vi "Subpanel - Load VI.vi"(7 "SubPanel in":refnum<vi>, 8 "error in (no error)":errorcluster, 10 "VI Reference":refnum<vi>, 11 "Subpanel VI Ref IN":refnum<vi>) -> (0 "error out":errorcluster, 2 "Removed Module":string, 3 "Subpanel VI Ref OUT":refnum<vi>)   [LabVIEW 2022 SP3, in "hse-ui.lvlib"]
doc: "Opens the VI reference to <b>Full Delimited Name</b> and inserts it into <b>SubPanel in</b>. The reference of the inserted VI is returned in Subpanel VI Ref OUT.\n\nIf Subpanel VI Ref IN is a valid reference, the front panel of the referenced VI is opened hidden before removing it from the subpanel in order to avoid losing the VI from memory.\n\n____\nHAMPEL SOFTWARE ENGINEERING v3.8.0 (2023-12-18 14:41)"
uses:
  hse-ui.lvlib
  hse-dqmh/hse-dqmh.lvlib
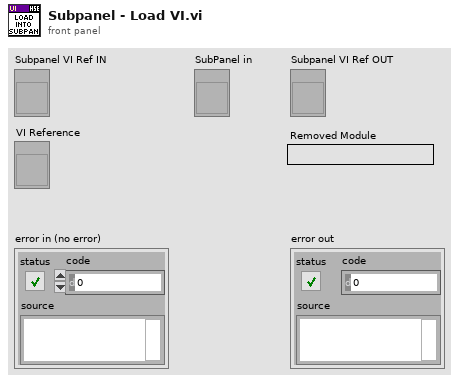
[diagram p1: front panel]
types:
  T1 = enum32{"Invalid", "Standard", "Closed", "Hidden", "Minimized", "Maximized"}
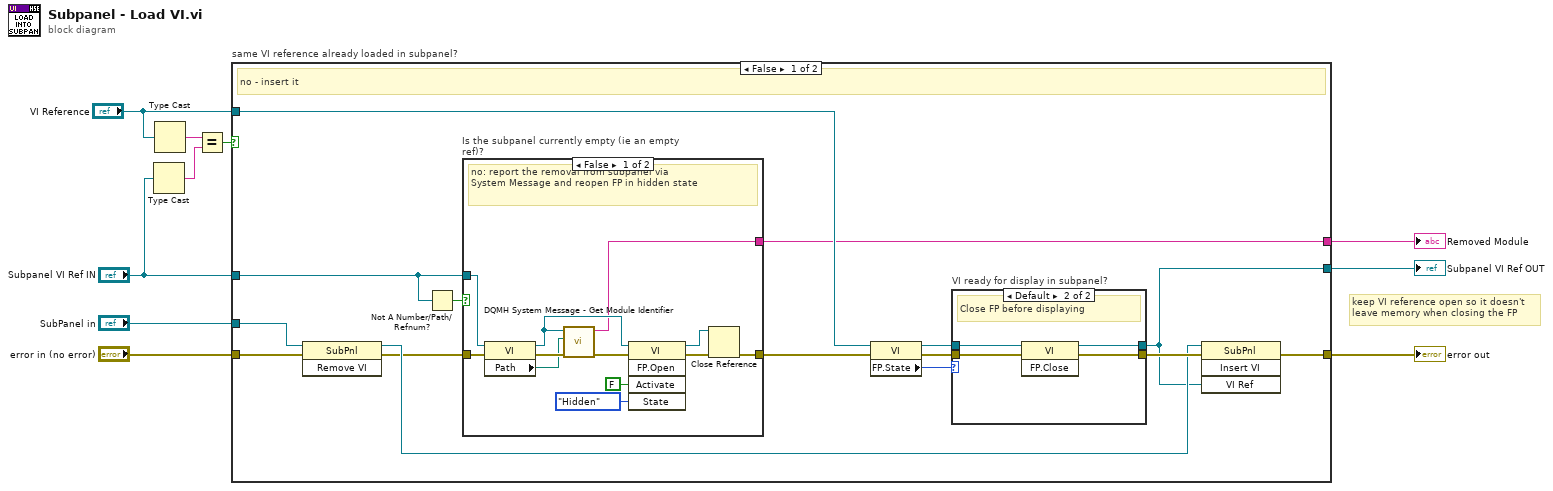
[diagram p0: block diagram]
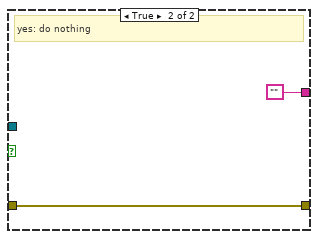
[diagram p2: hidden frame]
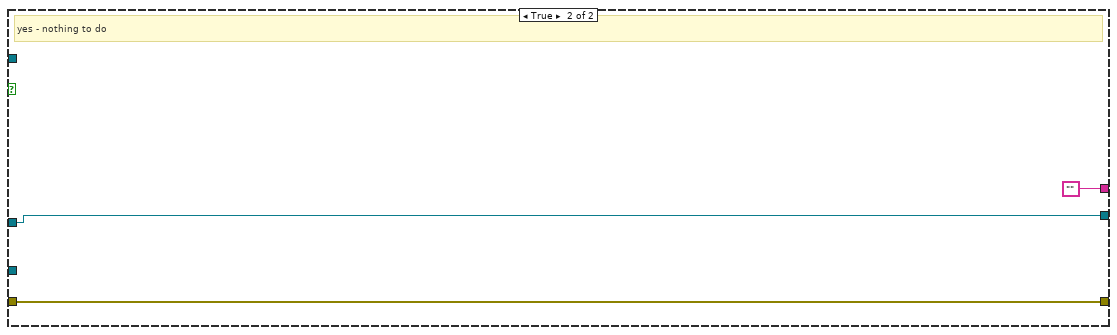
[diagram p4: hidden frame]
diagram:
  # "keep VI reference open so it doesn't\nleave memory when closing the FP"
  n1 = Type Cast(x="Subpanel VI Ref IN") -> (*(type *) &x=w2:string)  [unwired: 1 in]
  n2 = Type Cast(x="VI Reference") -> (*(type *) &x=w1:string)  [unwired: 1 in]
  n3 = Equal?(x=w1, y=w2) -> (x = y?=w5:bool)
  n4 = case "same VI reference already loaded in subpanel?" shown="False" w5 {
    tunnel: "error in (no error)" -> [w25 w46]
    tunnel: "SubPanel in" -> [w24 _]
    tunnel: [w18 w47] -> w9
    tunnel: [w17 w46] -> w8
    tunnel: "Subpanel VI Ref IN" -> [w15 w47]
    tunnel: "VI Reference" -> [w12 _]
    tunnel: [w11 ""] -> w7
    frame False {
      # "no - insert it"
      n5 = invoke on="Invoke Node" class="SubPnl" method="Remove VI"(reference=w24, error in=w25) -> (reference out=w20:refnum<vi>, error out=w16:errorcluster)  [unwired: 1 in, 1 out]
      n6 = Not A Number/Path/Refnum?(number/path/refnum=w15) -> (NaN/Path/Refnum?=w14:bool)
      n7 = case "Is the subpanel currently empty (ie an empty ref)?" shown="False" w14 {
        tunnel: w16 -> [w31 w39]
        tunnel: [w36 w39] -> w13
        tunnel: w15 -> [w32 _]
        tunnel: [w26 ""] -> w11
        frame False {
          # "no: report the removal from subpanel via \nSystem Message and reopen FP in hidden state"
          n8 = property class="VI"(reference=w32, error in=w31) -> (reference out=w27:refnum<vi>, error out=w30:errorcluster, "Path"=w28:path)
          n9 = call "DQMH System Message - Get Module Identifier.vi"("error in (no error)"=w30, "Module Path"=w28, "VI Ref"=w27) -> ("error out"=w29:errorcluster, "Module Identifier"=w26:string)  [unwired: 7 in]
          n10 = invoke on="Invoke Node" class="VI" method="FP.Open"(reference=w27, error in=w29, "Activate"=FALSE ("Activate?"), "State"=T1."Hidden") -> (reference out=w35:refnum<vi>, error out=w37:errorcluster)  [unwired: 1 in, 3 out]
          n11 = Close Reference(reference=w35, error in (no error)=w37) -> (error out=w36:errorcluster)
        }
        frame True {
          # "yes: do nothing"
        }
      }
      n12 = property class="VI"(reference=w12, error in=w13) -> (reference out=w23:refnum<vi>, error out=w22:errorcluster, "FP.State"=w19:T1)
      n13 = case "VI ready for display in subpanel?" shown="Default" w19 {
        tunnel: w23 -> [w41 w45]
        tunnel: w22 -> [w40 w44]
        tunnel: [w40 w43] -> w21
        tunnel: [w41 w42] -> w18
        frame "Invalid", "Closed" {
          # "state allows display in subpanel"
        }
        frame Default {
          # "Close FP before displaying"
          n14 = invoke on="Invoke Node" class="VI" method="FP.Close"(reference=w45, error in=w44) -> (reference out=w42:refnum<vi>, error out=w43:errorcluster)  [unwired: 1 in, 1 out]
        }
      }
      n15 = invoke on="Invoke Node" class="SubPnl" method="Insert VI"(reference=w20, error in=w21, "VI Ref"=w18) -> (error out=w17:errorcluster)  [unwired: 1 in, 3 out]
    }
    frame True {
      # "yes - nothing to do"
    }
  }
  "error out" <- w8
  "Subpanel VI Ref OUT" <- w9
  "Removed Module" <- w7
